vi "Fly.vi"(8 "error in (no error)":errorcluster, 11 "TurkeyAdapter in":refnum<class "TurkeyAdapter.lvclass">) -> (0 "error out":errorcluster, 2 "Fly":string, 3 "TurkeyAdapter out":refnum<class "TurkeyAdapter.lvclass">)   [LabVIEW 2013, in "TurkeyAdapter.lvclass"]
uses:
  TurkeyAdapter.lvclass
  TurkeyAdapter.lvclass/TurkeyAdapter.ctl
  Turkey.lvclass/Turkey.lvclass
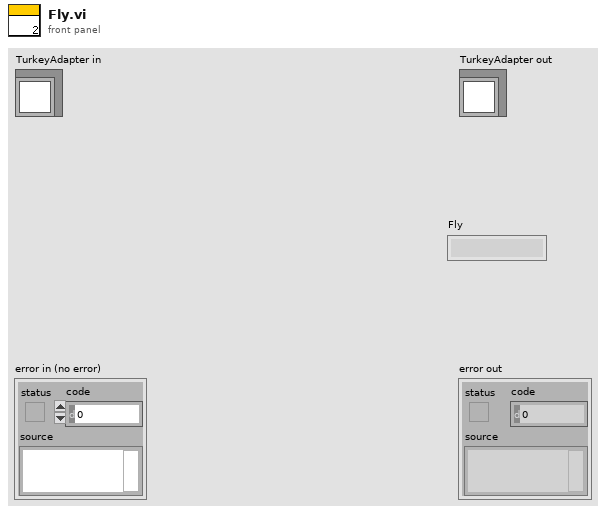
[diagram p1: front panel]
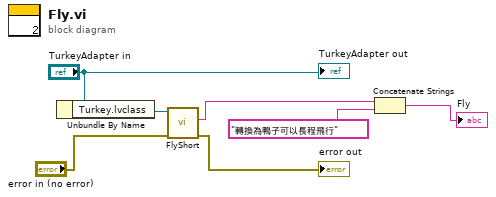
[diagram p0: block diagram]
diagram:
  n1 = Unbundle By Name("TurkeyAdapter in") -> ("Turkey.lvclass"=w4:refnum<class "Turkey.lvclass">)
  n2 = call-dynamic "FlyShort.vi"("error in (no error)"="error in (no error)", "Turkey in"=w4) -> ("error out"=→"error out":errorcluster, "Fiy"=w1:string)  [unwired: 7 in, 1 out]
  n3 = Concatenate Strings(w1, "轉換為鴨子可以長程飛行" ("string")) -> (→"Fly":string)
  "TurkeyAdapter out" <- "TurkeyAdapter in"
